vi "init.vi"(8 "error in (no error)":errorcluster, 11 "BoolUserEventStopMechanism In":refnum<class "BoolUETaskChannel.lvclass">) -> (0 "error out":errorcluster, 3 "BoolUserEventStopMechanism Out":refnum<class "BoolUETaskChannel.lvclass">)   [LabVIEW 2023, in "TLC_Daemon.lvlib" / "BoolUETaskChannel.lvclass"]
doc: "Initializes the Task Channel."
uses:
  BoolUETaskChannel/BoolUETaskChannel.lvclass
  BoolUETaskChannel/BoolUETaskChannel.lvclass/BoolUETaskChannel.ctl
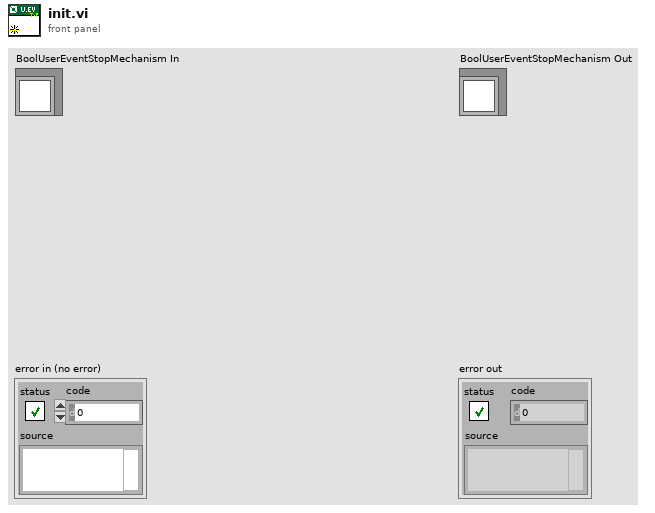
[diagram p1: front panel]
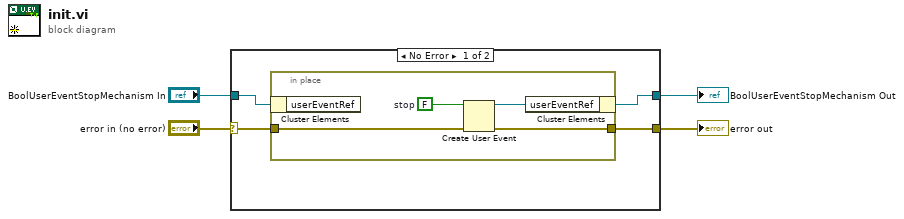
[diagram p0: block diagram]
diagram:
  n1 = case shown="No Error" "error in (no error)" {
    selector: "error in (no error)" -> [w8 w14]
    tunnel: [w7 w14] -> w4
    tunnel: [w5 w13] -> w1
    tunnel: "BoolUserEventStopMechanism In" -> [w6 w13]
    frame No Error {
      n2 = in-place {
        in-place-border: w8 -> [w11]
        in-place-border: [w10] -> w7
        w12 = FALSE  # stop
        n3 = in-place-cluster #1(w6) -> ()  [unwired: 1 out]
        n4 = Create User Event(user event datatype=w12, error in=w11) -> (user event=w9:refnum<user-event>, error out=w10:errorcluster)
        n5 = in-place-cluster #1("userEventRef"=w9) -> (w5:refnum<class "BoolUETaskChannel.lvclass">)
      }
    }
    frame Error {
    }
  }
  "error out" <- w4
  "BoolUserEventStopMechanism Out" <- w1
